vi "chart series set trendline.vi"(8 "error in (no error)":errorcluster, 9 "value":u8, 10 "type":u8, 11 "series":u32) -> (0 "error out":errorcluster)   [LabVIEW 8.6]
doc: "void chart_series_set_trendline(lxw_chart_series series, uint8_t type, uint8_t value);"
uses:
  pending_lvxlsxwriter/xlsxwriter.dll
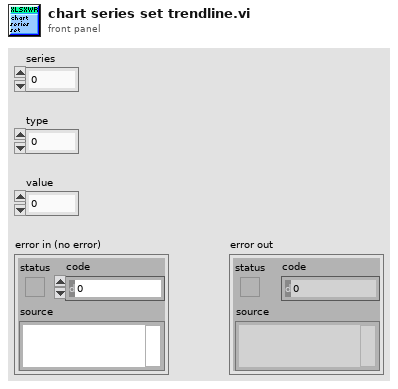
[diagram p1: front panel]
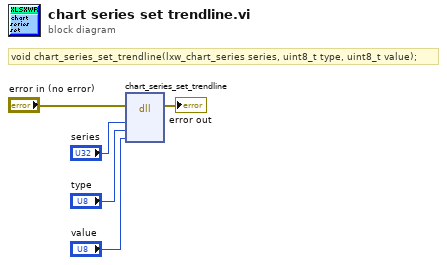
[diagram p0: block diagram]
diagram:
  # "void chart_series_set_trendline(lxw_chart_series series, uint8_t type, uint8_t value);"
  n1 = dll-call lib="C:/Users/WDAGUtilityAccount/Desktop/pending_lvxlsxwriter/xlsxwriter.*" fn="chart_series_set_trendline"(error in="error in (no error)", "series"="series", "type"="type", "value"="value") -> (error out=→"error out":errorcluster)  [unwired: 6 in, 1 out]
